vi "String as Encoded String (LabVIEW String).vi"(6 "error in":errorcluster, 9 "String":string) -> (1 "Encoded String":T1, 4 "error out":errorcluster)   [LabVIEW 2020, in "G-Unicode.lvlib"]
doc: "Converts the input string to a UTF-8 encoded LabVIEW string."
uses:
  G-Unicode.lvlib
  Types/Encoded UTF-8 String.ctl
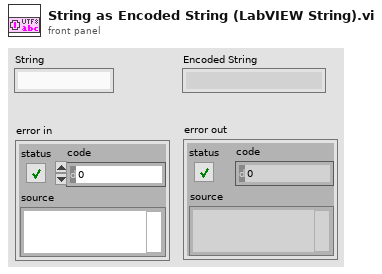
[diagram p1: front panel]
types:
  T1 = typedef "G-Unicode.lvlib/Encoded UTF-8 String.ctl" = string
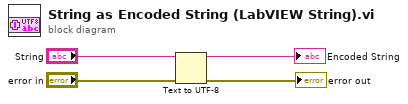
[diagram p0: block diagram]
diagram:
  n1 = Text to UTF-8(8:"error in", 11:"String") -> (0:→"error out":errorcluster, 3:→"Encoded String":string)  [unwired: 1 in]
